vi "Load Script.vi"(7 "Console Log in":refnum<class "Console Log.lvclass">, 8 "error in (no error)":errorcluster, 10 "Commands In":string[](array[string]), 11 "gScript Interpreter in":refnum<class "gScript Interpreter.lvclass">) -> (0 "error out":errorcluster, 3 "gScript Interpreter out":refnum<class "gScript Interpreter.lvclass">, 5 "Console Log out":refnum<class "Console Log.lvclass">)   [LabVIEW 2017, in "gScript Interpreter.lvclass"]
uses:
  gScript Interpreter.lvclass
  Application Utilities/Console Log/Console Log.lvclass
  Type Definitions/Label.ctl
  gScript Interpreter.lvclass/gScript Interpreter.ctl
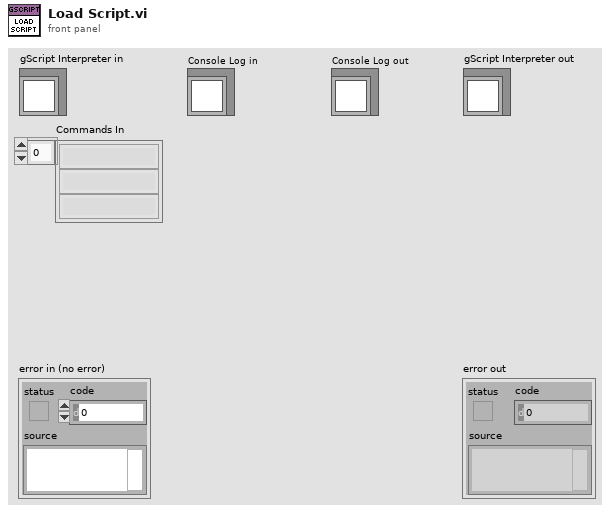
[diagram p1: front panel]
types:
  T1 = typedef "Label.ctl" = cluster{"Label":string, "Line":i32, "Arguments":string[]}
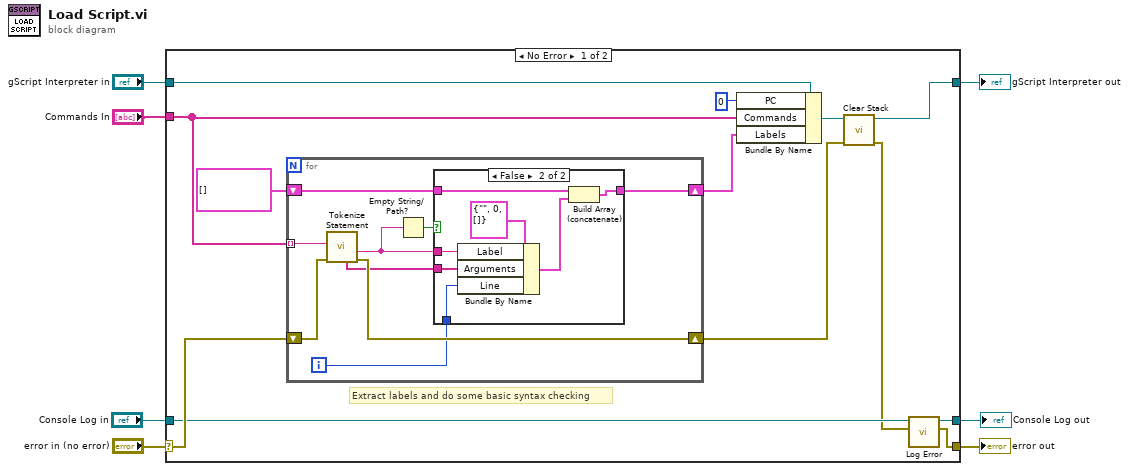
[diagram p0: block diagram]
diagram:
  n1 = case shown="No Error" "error in (no error)" {
    selector: "error in (no error)" -> [w18 w40]
    tunnel: [w13 w40] -> w6
    tunnel: [w10 w39] -> w4
    tunnel: "gScript Interpreter in" -> [w20 w39]
    tunnel: "Commands In" -> [w16 _]
    tunnel: "Console Log in" -> [w15 w38]
    tunnel: [w14 w38] -> w1
    frame No Error {
      # "Extract labels and do some basic syntax checking"
      n2 = for {
        tunnel: w16 -> [w29] mode=indexing
        shift-right: [w25] -> w17
        shift-left: T1[] [] -> [w26]
        shift-right: [w27] -> w9
        shift-left: w18 -> [w28]
        i -> [w24]
        n3 = call "Tokenize Statement.vi"("error in (no error)"=w28, "Command"=w29) -> ("error out"=w27:errorcluster, "Label"=w23:string, "Label Arguments"=w21:string[])  [unwired: 5 in, 2 out]
        n4 = Empty String/Path?(string/path=w23) -> (empty?=w22:bool)
        n5 = case shown="False" w22 {
          tunnel: w23 -> [_ w37]
          tunnel: w26 -> [w30 w36]
          tunnel: [w30 w34] -> w25
          tunnel: w24 -> [_ w33]
          tunnel: w21 -> [_ w31]
          frame True {
          }
          frame False {
            n6 = Bundle By Name(cluster=T1 {"Label"="", "Line"=0, "Arguments"=[]} ("Label"), "Label"=w37, "Arguments"=w31, "Line"=w33) -> (w35:T1)
            n7 = Build Array (concatenate)(w36, w35) -> (w34:T1[])
          }
        }
      }
      n8 = Bundle By Name(cluster=w20, "PC"=0, "Commands"=w16, "Labels"=w17) -> (w11:refnum<class "gScript Interpreter.lvclass">)
      n9 = call "Clear Stack.vi"("error in (no error)"=w9, "gScript Interpreter in"=w11) -> ("error out"=w8:errorcluster, "gScript Interpreter out"=w10:refnum<class "gScript Interpreter.lvclass">)  [unwired: 8 in]
      n10 = call "Log Error.vi"("error in"=w8, "Console Log in"=w15) -> ("error out"=w13:errorcluster, "Console Log out"=w14:refnum<class "Console Log.lvclass">)  [unwired: 8 in]
    }
    frame Error {
    }
  }
  "error out" <- w6
  "gScript Interpreter out" <- w4
  "Console Log out" <- w1
